vi "XY Heading to Bearing.vi"(1 "XY Heading (Degrees)":dbl) -> (0 "Bearing (Degrees from North CW)":dbl)   [LabVIEW 2009]
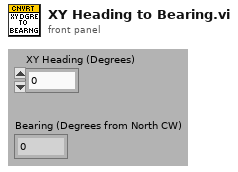
[diagram p1: front panel]
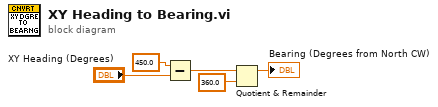
[diagram p0: block diagram]
diagram:
  n1 = Subtract(x=450.0, y="XY Heading (Degrees)") -> (x-y=w3:dbl)
  n2 = Quotient & Remainder(x=w3, y=360.0) -> (x-y*floor(x/y)=→"Bearing (Degrees from North CW)":dbl)  [unwired: 1 out]
